vi "toJSON.vi"(8 "error in (no error)":errorcluster, 11 "tBSONString in":refnum<class "tBSONString.lvclass">) -> (0 "error out":errorcluster, 2 "JSON":string, 3 "tBSONString out":refnum<class "tBSONString.lvclass">)   [LabVIEW 2013, in "BSON.lvlib" / "tBSONString.lvclass"]
uses:
  tBSONString.lvclass
  tBSONElement/tBSONElement.lvclass
  getValue.vi
  BSON.lvlib
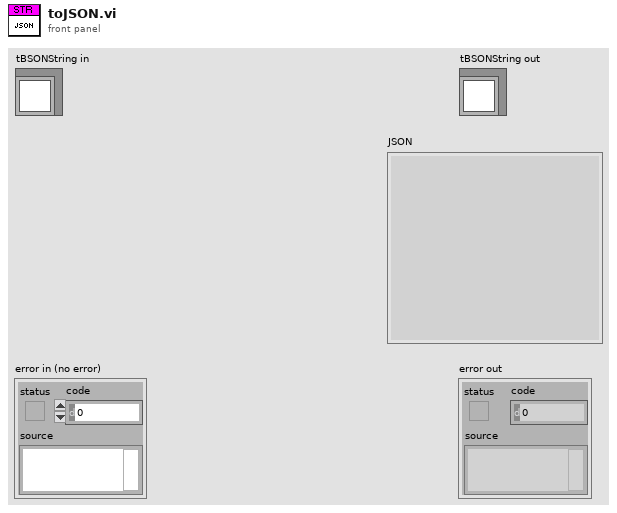
[diagram p1: front panel]
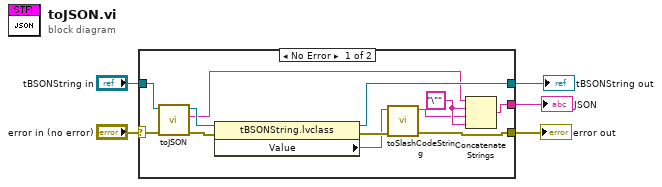
[diagram p0: block diagram]
diagram:
  n1 = case shown="No Error" "error in (no error)" {
    selector: "error in (no error)" -> [w17 w18]
    tunnel: "tBSONString in" -> [w16 w19]
    tunnel: [w13 w19] -> w3
    tunnel: [w6 w18] -> w2
    tunnel: [w12 _] -> w1
    frame No Error {
      w10 = "\"" ("string")
      n2 = call-parent "toJSON.vi"("error in (no error)"=w17, "tBSONElement in"=w16) -> ("error out"=w14:errorcluster, "JSON"=w11:string, "tBSONElement out"=w15:refnum<class "tBSONString.lvclass">)  [unwired: 7 in]
      n3 = property class="tBSONString.lvclass"(reference=w15, error in=w14) -> (reference out=w13:refnum<class "tBSONString.lvclass">, error out=w9:errorcluster, "Value"=w8:string)
      n4 = call "toSlashCodeString.vi"("error in (no error)"=w9, "String In"=w8) -> ("error out"=w6:errorcluster, "String Out"=w7:string)  [unwired: 8 in]
      n5 = Concatenate Strings(w11, w10, w7, w10) -> (w12:string)
    }
    frame Error {
    }
  }
  "error out" <- w2
  "tBSONString out" <- w3
  "JSON" <- w1
